vi "MoveAbsolute (units).vi"(7 "Wait Timeout, ms (60000)":i32=60000, 8 "error in (no error)":errorcluster, 9 "Y, units":dbl, 10 "X, units":dbl, 11 "XYStage":refnum<class "XYStage.lvclass">) -> (0 "error out":errorcluster, 3 "XYStage out":refnum<class "XYStage.lvclass">)   [LabVIEW 2017, in "XYStage.lvclass"]
doc: "---------------------------------------------------------------\nJKI State Machine Objects™\nhttp://jki.net/state-machine-objects/\nCopyright (C) 2005-2015, JKI <info@jki.net>\nALL RIGHTS RESERVEDJKI State Machine Objects (SMO) 1.0.0.4\nJKI - JKI\nCopyright (c) 2015, JKI"
uses:
  XYStage.lvclass
  Typedefs/PrivateEvents--XYStage.MoveAbsolute (units).ctl
  Typedefs/Coordinates.Units--Cluster.ctl
  XYStage.lvclass/XYStage.ctl
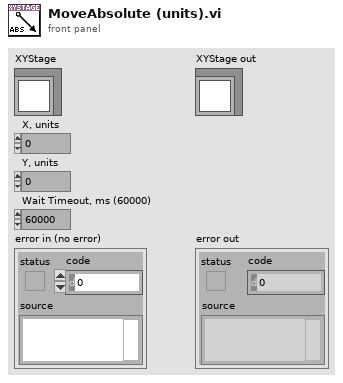
[diagram p1: front panel]
types:
  T1 = typedef "XYStage.lvclass/PrivateEvents--XYStage.MoveAbsolute (units).ctl" = cluster{"Coordinates.Units":T2, "Wait Timeout, ms":i32}
  T2 = typedef "XYStage.lvclass/Coordinates.Units--Cluster.ctl" = cluster{"X":dbl, "Y":dbl}
  T3 = typedef "XYStage.lvclass/PrivateData--Ref.ctl" = refnum<data-value>
  T4 = typedef "XYStage.lvclass/PrivateData--Cluster.ctl" = cluster{"Configuration":T5, "Public Events":T6, "Protected Events":T7, "Private Events":T8}
  T5 = typedef "XYStage.lvclass/Configuration--Cluster.ctl" = cluster{"Serial Number":string, "X Axis":string, "Y Axis":string, "Real-World Units":string, "Counts per Unit":u32}
  T6 = typedef "XYStage.lvclass/PublicEvents--Cluster.ctl" = cluster{"MoveStarted":refnum<user-event>, "MoveCompleted":refnum<user-event>}
  T7 = typedef "XYStage.lvclass/ProtectedEvents--Cluster.ctl" = cluster{"StatusUpdated":refnum<user-event>}
  T8 = typedef "XYStage.lvclass/PrivateEvents--Cluster.ctl" = cluster{"MoveAbsolute (units)":refnum<user-event>}
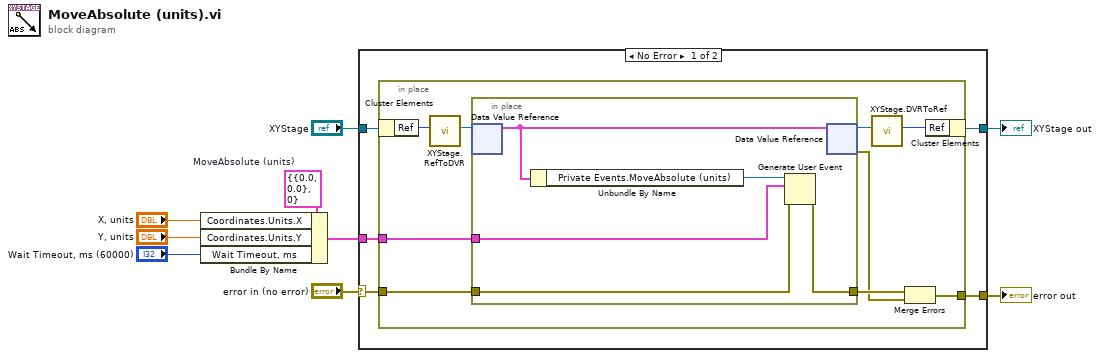
[diagram p0: block diagram]
diagram:
  w5 = T1 {"Coordinates.Units"={"X"=0.0, "Y"=0.0}, "Wait Timeout, ms"=0}  # MoveAbsolute (units)
  n1 = Bundle By Name(cluster=w5, "Coordinates.Units.X"="X, units", "Coordinates.Units.Y"="Y, units", "Wait Timeout, ms"="Wait Timeout, ms (60000)") -> (w1:T1)
  n2 = case shown="No Error" "error in (no error)" {
    selector: "error in (no error)" -> [w12 w30]
    tunnel: [w11 w30] -> w8
    tunnel: [w13 w29] -> w9
    tunnel: "XYStage" -> [w14 w29]
    tunnel: w1 -> [w10 _]
    frame No Error {
      n3 = in-place {
        in-place-border: w12 -> [w23]
        in-place-border: [w15] -> w11
        in-place-border: w10 -> [w18]
        n4 = in-place-cluster #1(w14) -> ("Ref"=w20:u32)
        n5 = call "XYStage.RefToDVR.vi"("Ref"=w20) -> ("Ref"=w17:T3)  [unwired: 10 in]
        n6 = in-place {
          in-place-border: w23 -> [w26]
          in-place-border: [w25] -> w22
          in-place-border: w18 -> [w24]
          n7 = in-place-dvr #2(w17) -> (w28:T4)  [unwired: 1 out]
          n8 = Unbundle By Name(w28) -> ("Private Events.MoveAbsolute (units)"=w27:refnum<user-event>)
          n9 = Generate User Event(user event=w27, event data cluster=w24, error in=w26) -> (error out=w25:errorcluster)  [unwired: 1 in, 1 out]
          n10 = in-place-dvr #2(w28) -> (w19:T3, w21:errorcluster)
        }
        n11 = call "XYStage.DVRToRef.vi"("Ref"=w19) -> ("Ref"=w16:u32)  [unwired: 10 in]
        n12 = Merge Errors(w22, w21) -> (w15:errorcluster)
        n13 = in-place-cluster #1("Ref"=w16) -> (w13:refnum<class "XYStage.lvclass">)
      }
    }
    frame Error {
    }
  }
  "error out" <- w8
  "XYStage out" <- w9
